vi "Bin Array.vi"(10 "#bins":i32, 11 "Array":dbl[](array[numeric])) -> (3 "Binned array":dbl[](array[numeric]))   [LabVIEW 2013]
uses:
  <vilib>/Analysis/2dsp.llb/Zero Padder (DBL).vi
  <vilib>/Analysis/NI_AALPro.lvlib
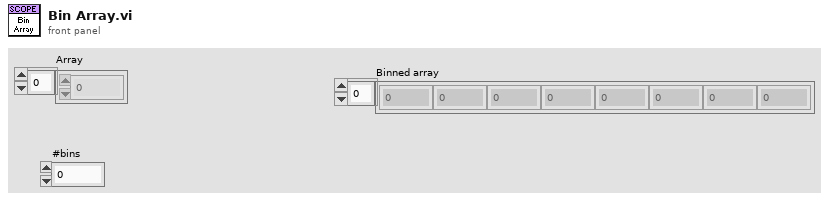
[diagram p1: front panel]
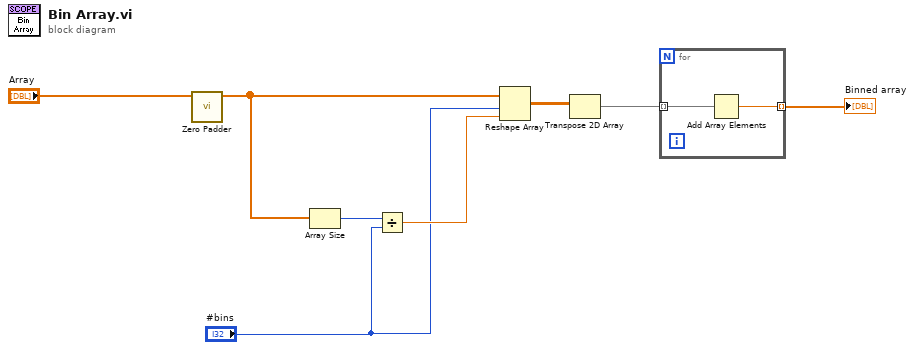
[diagram p0: block diagram]
diagram:
  n1 = call-poly <vilib>:"Zero Padder.vi"("Input Array"="Array") -> ("Zero Padded Array"=w1:dbl[])  [unwired: 10 in]
  n2 = Array Size(array=w1) -> (size(s)=w8:i32)
  n3 = Divide(x=w8, y="#bins") -> (x/y=w7:dbl)
  n4 = Reshape Array(w1, "#bins", w7) -> (w2:dbl[][])
  n5 = Transpose 2D Array(2D array=w2) -> (transposed array=w4:dbl[][])
  n6 = for {
    tunnel: w4 -> [w10] mode=indexing
    tunnel: [w9] -> w5 mode=indexing
    n7 = Add Array Elements(numeric array=w10) -> (sum=w9:dbl)
  }
  "Binned array" <- w5
